vi "Write Element of STRANS.vi"(8 "error in (no error)":errorcluster, 9 "Bit":bool, 10 "index":i32, 11 "Referential in":refnum<class "Referential.lvclass">) -> (0 "error out":errorcluster, 3 "Referential out":refnum<class "Referential.lvclass">)   [LabVIEW 2019, in "Referential.lvclass"]
uses:
  Referential.lvclass
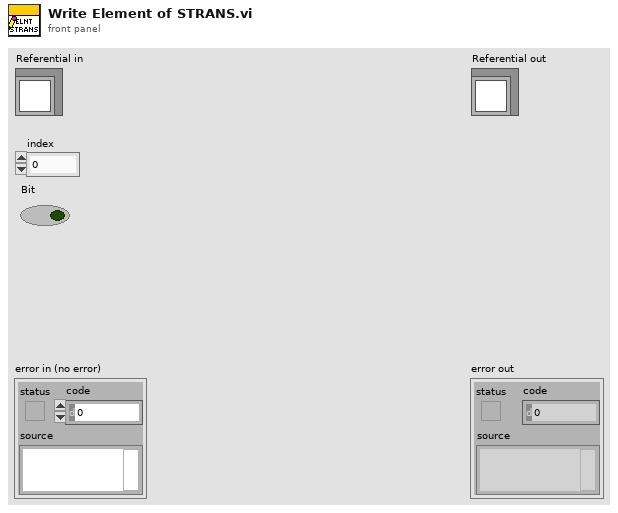
[diagram p1: front panel]
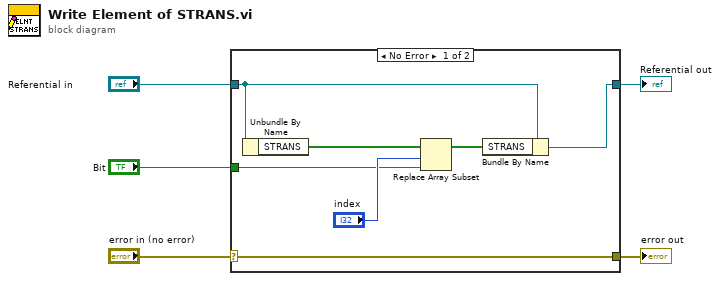
[diagram p0: block diagram]
diagram:
  n1 = case shown="No Error" "error in (no error)" {
    selector: "error in (no error)" -> [w12 w13]
    tunnel: [w12 w13] -> w4
    tunnel: [w11 w14] -> w2
    tunnel: "Referential in" -> [w10 w14]
    tunnel: "Bit" -> [w6 _]
    frame No Error {
      n2 = Unbundle By Name(w10) -> ("STRANS"=w9:bool[])
      n3 = Replace Array Subset(array=w9, new element=w6, index="index") -> (w8:bool[])
      n4 = Bundle By Name(cluster=w10, "STRANS"=w8) -> (w11:refnum<class "Referential.lvclass">)
    }
    frame Error {
    }
  }
  "error out" <- w4
  "Referential out" <- w2
